vi "DB Open.vi"(8 "error in":errorcluster, 10 "DB":T1={"DataSource Name"="eDCU_LTT", "userID"="root", "password"="edultt"}, 11 "Database in":refnum<class "MYSQL Server.lvclass">) -> (0 "error out":errorcluster, 3 "Database out":refnum<class "MYSQL Server.lvclass">)   [LabVIEW 2023, in "HardwareAbstractionLayer_LVOOP.lvlib" / "MYSQL Server.lvclass"]
doc: "This VI is Database Connection Open"
uses:
  MYSQL Server.lvclass
  MYSQL Server.lvclass/MYSQL Server.ctl
  <vilib>/addons/database/Connection.llb/DB Tools Open Connec (String).vi
  <vilib>/addons/database/NI_Database_API.lvlib
  Database.lvclass
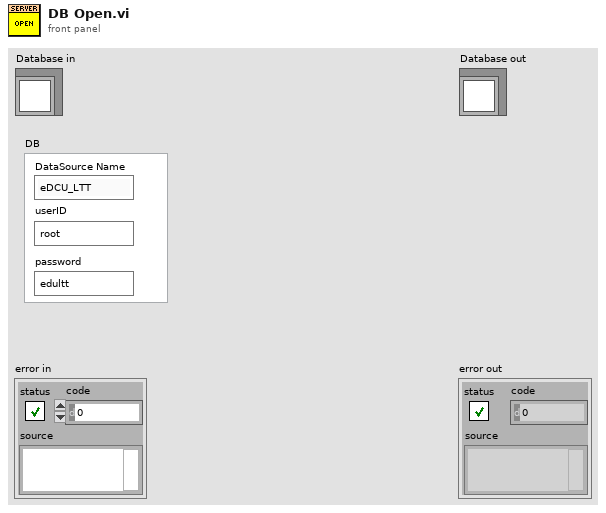
[diagram p1: front panel]
types:
  T1 = cluster{"DataSource Name":string, "userID":string, "password":string}
  T2 = typedef "NI_Database_API.lvlib/Conn ObjectReference.ctl" = refnum<k1>
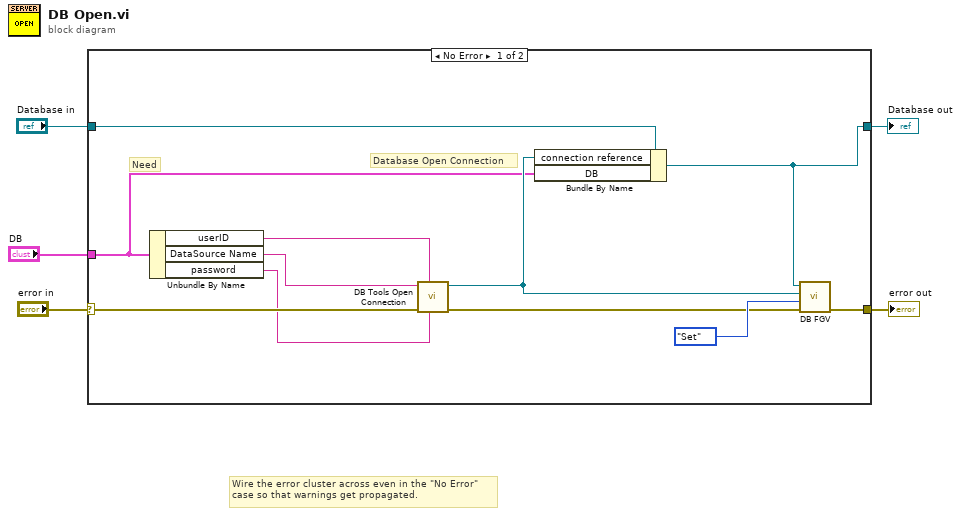
[diagram p0: block diagram]
diagram:
  # "Wire the error cluster across even in the \"No Error\"\ncase so that warnings get propagated."
  n1 = case shown="No Error" "error in" {
    selector: "error in" -> [w16 w18]
    tunnel: [w9 w18] -> w4
    tunnel: [w8 w17] -> w2
    tunnel: "Database in" -> [w12 w17]
    tunnel: "DB" -> [w6 _]
    frame No Error {
      # "Need"
      # "Database Open Connection"
      n2 = Unbundle By Name(w6) -> ("userID"=w15:string, "DataSource Name"=w14:string, "password"=w13:string)
      n3 = call-poly <vilib>:"DB Tools Open Connection.vi"("password"=w13, "userID"=w15, "error in (no error)"=w16, "connection information"=w14) -> ("error out"=w10:errorcluster, "connection reference"=w7:T2)  [unwired: 4 in]
      n4 = Bundle By Name(cluster=w12, "connection reference"=w7, "DB"=w6) -> (w8:refnum<class "MYSQL Server.lvclass">)
      n5 = call "DB FGV.vi"("error in"=w10, "Action"=enum16{"Get", "Set"}."Set", "connection reference"=w7, "Database.lvclass"=w8) -> ("error out"=w9:errorcluster)  [unwired: 5 in, 2 out]
    }
    frame Error {
    }
  }
  "error out" <- w4
  "Database out" <- w2
